vi "Stop Streaming.vi"(8 "error in (no error)":errorcluster, 11 "Synchronization Device in":refnum<class "Microsync.lvclass">) -> (0 "error out":errorcluster, 3 "Synchronization Device out":refnum<class "Microsync.lvclass">)   [LabVIEW 2023, in "Microsync.lvlib" / "Microsync.lvclass"]
uses:
  Microsync.lvclass
  Microsync.lvclass/Microsync.ctl
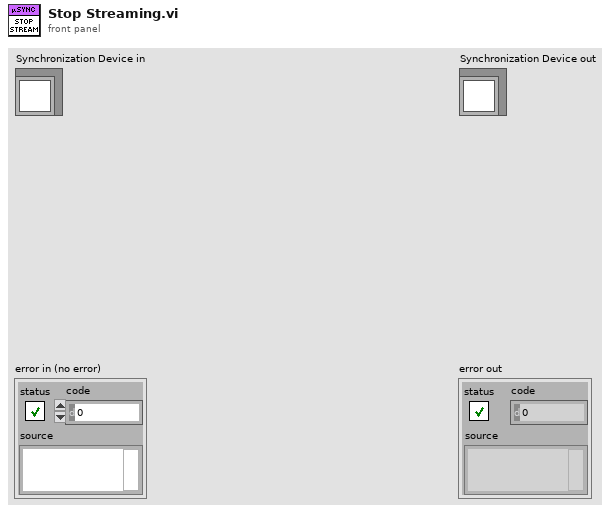
[diagram p1: front panel]
types:
  T1 = enum16{"ro_VERSION", "ro_SYS_TIMER_STATUS", "ro_SYS_TIMER_VALUE", "ro_SYS_TIMER_OVF_COUNT", "ro_SYS_TIME_ms", "ro_SYS_TIMER_PRESCALER", "rw_DFLT_PULSE_DURATION_us", "ro_WATCHDOG_TIMEOUT_ms", "ro_N_EVENTS", "rw_INTLCK_ENABLED", "rw_SELECTED_LASERS", "wo_OPEN_SHUTTERS", "wo_CLOSE_SHUTTERS", "rw_SHUTTER_DELAY_us", "rw_CAM_READOUT_us"}
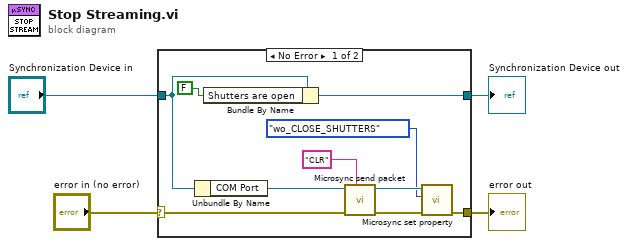
[diagram p0: block diagram]
diagram:
  n1 = case shown="No Error" "error in (no error)" {
    selector: "error in (no error)" -> [w13 w16]
    tunnel: "Synchronization Device in" -> [w7 w15]
    tunnel: [w5 w15] -> w2
    tunnel: [w11 w16] -> w1
    frame No Error {
      n2 = Unbundle By Name(w7) -> ("COM Port"=w12:refnum<visa-resource-name>)
      n3 = Bundle By Name(cluster=w7, "Shutters are open"=FALSE) -> (w5:refnum<class "Microsync.lvclass">)
      n4 = call "Microsync send packet.vi"("Command"="CLR", "error in (no error)"=w13, "VISA resource name"=w12) -> ("error out"=w10:errorcluster, "VISA resource name out"=w9:refnum<visa-resource-name>)  [unwired: 6 in, 1 out]
      n5 = call "Microsync set property.vi"("error in (no error)"=w10, "property to set"=T1."wo_CLOSE_SHUTTERS", "VISA resource name"=w9) -> ("error out"=w11:errorcluster)  [unwired: 7 in, 1 out]
    }
    frame Error {
    }
  }
  "error out" <- w1
  "Synchronization Device out" <- w2
